vi "extract NOT RECD customer data.vi"(6 "File Path in":path, 9 "select source":enum32{"user selectable", "constant"}(ring), 11 "select cust":string) -> (0 "cyl list":string[](array[string]), 1 "cust list":string[](array[string]), 3 "cust data":string[][](array[string]))   [LabVIEW 2011]
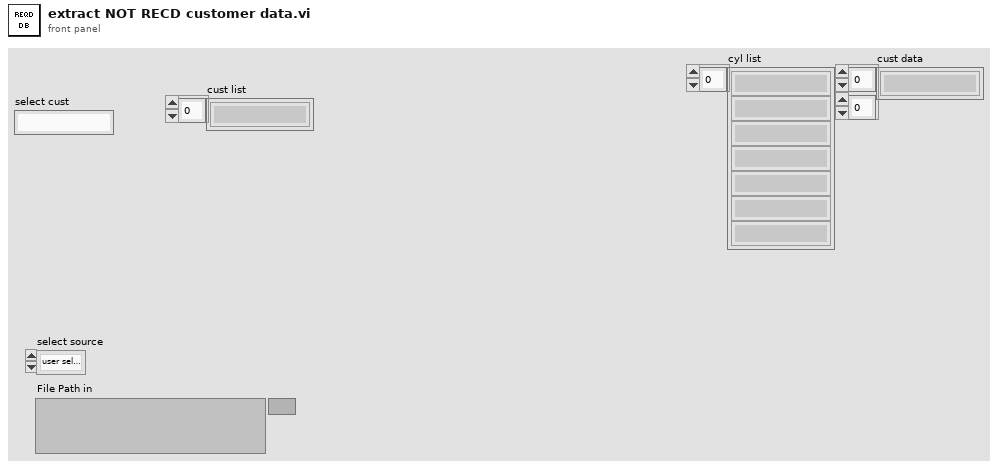
[diagram p1: front panel]
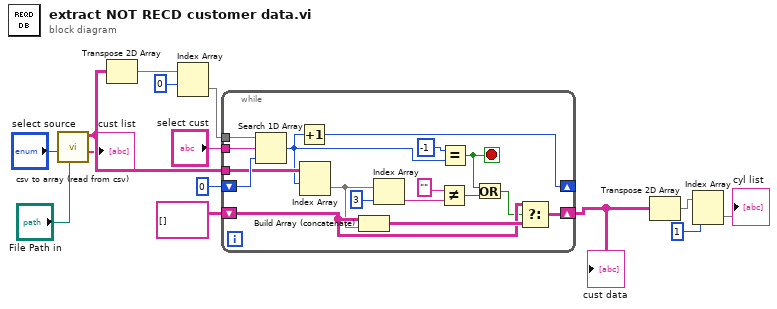
[diagram p0: block diagram]
diagram:
  n1 = call "csv to array (read from csv).vi"("File Path in"="File Path in", "select source"="select source") -> ("Array"=→"cust list":string[], "all rows"=w10:string[][])  [unwired: 8 in]
  n2 = Transpose 2D Array(2D array=w10) -> (transposed array=w13:string[][])
  n3 = Index Array(array=w13, index (row)=0) -> (element=w9:string[])  [unwired: 1 in]
  n4 = while {
    tunnel: w10 -> [w28]
    tunnel: "select cust" -> [w31]
    shift-right: [w27] -> _
    shift-left: 0 ("index of element") -> [w30]
    tunnel: w9 -> [w29]
    shift-right: [w23] -> w5
    shift-left: string[][] [] -> [w22]
    stop <- w15 stop-if-true
    n5 = Search 1D Array(1D array=w29, element=w31, start index (0)=w30) -> (index of element=w26:i32)
    n6 = Increment(x=w26) -> (x+1=w27:i32)
    n7 = Index Array(array=w28, index (row)=w26) -> (element=w21:string[])  [unwired: 1 in]
    n8 = Build Array (concatenate)(w22, w21) -> (w24:string[][])
    n9 = Index Array(array=w21, index=3) -> (element=w19:string)
    n10 = Not Equal?(x="", y=w19) -> (x != y?=w17:bool)
    n11 = Equal?(x=-1, y=w26) -> (x = y?=w15:bool)
    n12 = Or(x=w15, y=w17) -> (x .or. y?=w16:bool)
    n13 = Select(t=w22, s=w16, f=w24) -> (s? t:f=w23:string[][])
  }
  "cust data" <- w5
  n14 = Transpose 2D Array(2D array=w5) -> (transposed array=w6:string[][])
  n15 = Index Array(array=w6, index (row)=1) -> (element=→"cyl list":string[])  [unwired: 1 in]
